vi "shoot message.vi"(9 "shoot self":bool, 10 "P1 Turn":bool) -> (2 "String":string)   [LabVIEW 2025]
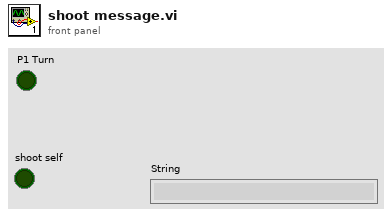
[diagram p1: front panel]
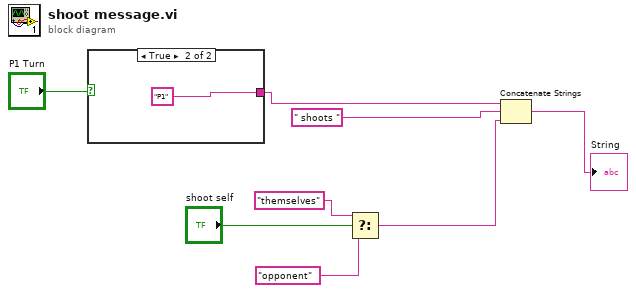
[diagram p0: block diagram]
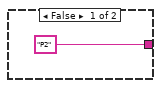
[diagram p2: hidden frame]
diagram:
  n1 = case shown="True" "P1 Turn" {
    tunnel: ["P2" "P1"] -> w7
    frame False {
    }
    frame True {
    }
  }
  n2 = Select(t="themselves", s="shoot self", f="opponent") -> (s? t:f=w2:string)
  n3 = Concatenate Strings(w7, " shoots ", w2) -> (→"String":string)
